vi "Async Rx.vi"(8 "error in (no error)":errorcluster, 9 "framework iteration":u64, 10 "Dispatcher Interface in":refnum<class "Dispatcher Interface.lvclass">, 11 "Plugin Timing Group in":refnum<class "Plugin Timing Group.lvclass">) -> (0 "error out":errorcluster, 2 "Dispatcher Interface out":refnum<class "Dispatcher Interface.lvclass">, 3 "Plugin Timing Group out":refnum<class "Plugin Timing Group.lvclass">)   [LabVIEW 2017, in "DSF Core.lvlib" / "Plugin Timing Group.lvclass"]
uses:
  Timing/Plugin Timing Group.lvclass
  Interfaces/Dispatcher/Dispatcher Interface.lvclass
  Timing/Plugin Timing Group.lvclass/Plugin Timing Group.ctl
  Timing/Timing.lvclass/Timing.ctl
  Timing/Get Decimation.vi
  Timing/Get Offset.vi
  Timing/Timing.lvclass
  Timing/Transfer Group Timing.lvclass
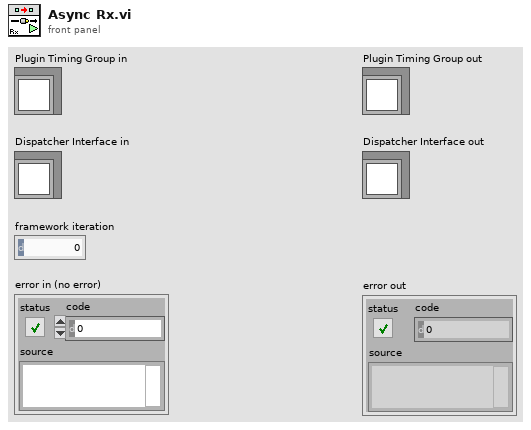
[diagram p1: front panel]
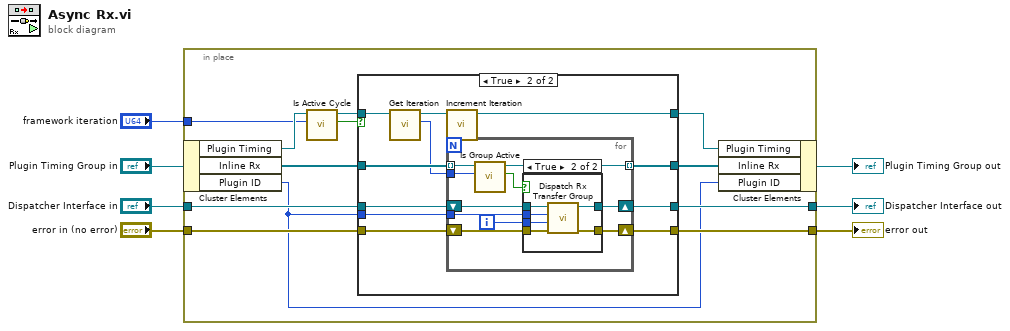
[diagram p0: block diagram]
diagram:
  n1 = in-place {
    in-place-border: "framework iteration" -> [w13]
    in-place-border: "Dispatcher Interface in" -> [w12]
    in-place-border: [w11] -> w4
    in-place-border: [w10] -> w2
    in-place-border: "error in (no error)" -> [w9]
    n2 = in-place-cluster #1("Plugin Timing Group in") -> ("Plugin Timing"=w15:refnum<class "Timing.lvclass">, "Inline Rx"=w19:refnum<class "Transfer Group Timing.lvclass">[], "Plugin ID"=w8:i32)
    n3 = call "Is Active Cycle.vi"("iteration"=w13, "Timing in"=w15) -> ("active?"=w17:bool, "Timing out"=w16:refnum<class "Timing.lvclass">)  [unwired: 8 in]
    n4 = case shown="True" w17 {
      tunnel: w19 -> [w23 w25]
      tunnel: [w23 w34] -> w18
      tunnel: w16 -> [w22 w33]
      tunnel: [w22 w26] -> w14
      tunnel: w12 -> [w21 w31]
      tunnel: [w21 w30] -> w11
      tunnel: [w20 w29] -> w10
      tunnel: w8 -> [_ w28]
      tunnel: w9 -> [w20 w27]
      frame False {
      }
      frame True {
        n5 = call "Get Iteration.vi"("Timing in"=w33) -> ("Iteration"=w24:u64, "Timing out"=w32:refnum<class "Timing.lvclass">)  [unwired: 9 in]
        n6 = call "Increment Iteration.vi"("Timing in"=w32) -> ("Timing out"=w26:refnum<class "Timing.lvclass">)  [unwired: 10 in]
        n7 = for {
          tunnel: w25 -> [w38] mode=indexing
          tunnel: [w36] -> w34 mode=indexing
          tunnel: w24 -> [w37]
          shift-right: [w43] -> w30
          shift-left: w31 -> [w44]
          shift-right: [w42] -> w29
          shift-left: w27 -> [w41]
          tunnel: w28 -> [w40]
          i -> [w39]
          n8 = call "Is Group Active.vi"("plugin iteration"=w37, "Transfer Group Timing in"=w38) -> ("active?"=w35:bool, "Transfer Group Timing out"=w36:refnum<class "Transfer Group Timing.lvclass">)  [unwired: 7 in, 1 out]
          n9 = case shown="True" w35 {
            tunnel: w44 -> [w46 w52]
            tunnel: [w46 w51] -> w43
            tunnel: [w45 w50] -> w42
            tunnel: w41 -> [w45 w49]
            tunnel: w40 -> [_ w48]
            tunnel: w39 -> [_ w47]
            frame False {
            }
            frame True {
              n10 = call "Dispatch Rx Transfer Group.vi"("error in (no error)"=w49, "Transfer Group ID"=w47, "Plugin ID"=w48, "Dispatcher Interface in"=w52) -> ("error out"=w50:errorcluster, "Dispatcher Interface out"=w51:refnum<class "Dispatcher Interface.lvclass">)  [unwired: 6 in]
            }
          }
        }
      }
    }
    n11 = in-place-cluster #1("Plugin Timing"=w14, "Inline Rx"=w18, "Plugin ID"=w8) -> (→"Plugin Timing Group out":refnum<class "Plugin Timing Group.lvclass">)
  }
  "Dispatcher Interface out" <- w4
  "error out" <- w2
